vi "02T_WaitForData.vi"(8 "WaitTimeoutMS":u32, 11 "VISA":refnum<visa-resource-name>) -> (0 "Buffer":string, 1 "Bytes at Port":u32, 3 "Data Recived":bool=TRUE)   [LabVIEW 2013]
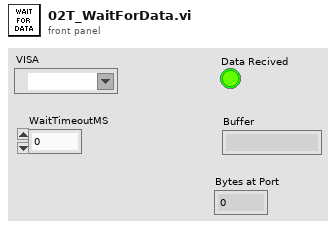
[diagram p1: front panel]
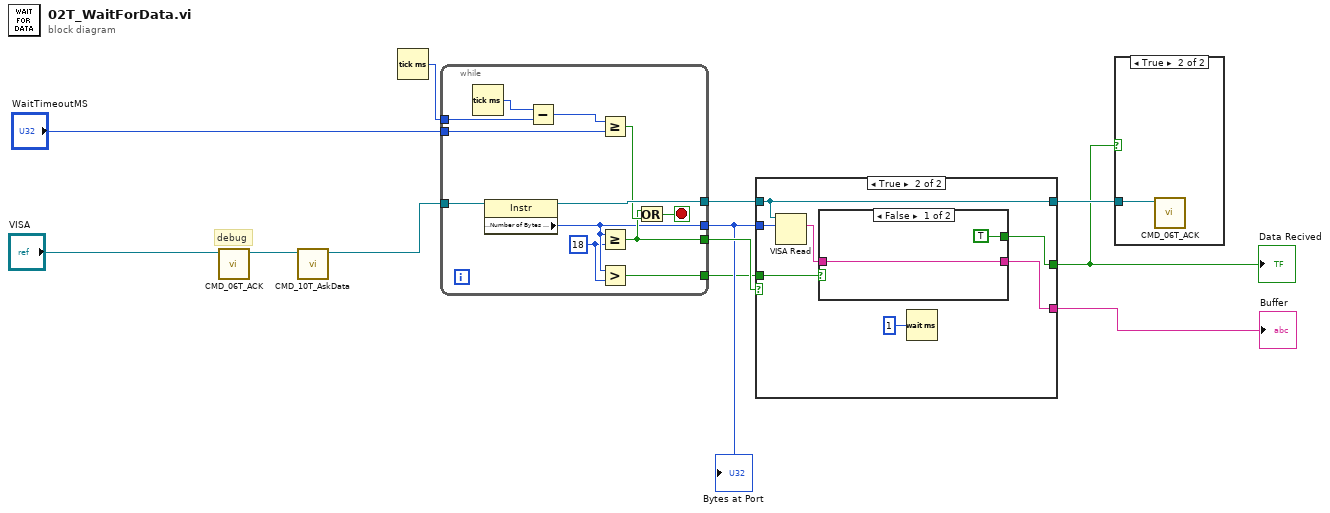
[diagram p0: block diagram]
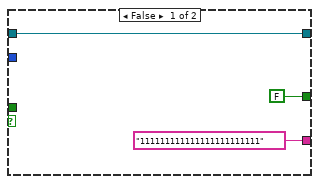
[diagram p3: hidden frame]
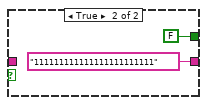
[diagram p4: hidden frame]
diagram:
  # "debug"
  n1 = call "CMD_06T_ACK.vi"("VISA resource name"="VISA") -> ("VISA resource name out"=w1:refnum<visa-resource-name>)  [unwired: 10 in]
  n2 = call "CMD_10T_AskData.vi"("VISA resource name"=w1) -> ("VISA resource name out"=w2:refnum<visa-resource-name>)  [unwired: 10 in]
  n3 = Tick Count (ms)() -> (millisecond timer value=w12:u32)
  n4 = while {
    tunnel: w2 -> [w24]
    tunnel: [w23] -> w9
    tunnel: [w15] -> w8
    tunnel: w12 -> [w20]
    tunnel: "WaitTimeoutMS" -> [w17]
    tunnel: [w16] -> w10
    tunnel: [w13] -> w7
    stop <- w22 stop-if-true
    w14 = u32 18 ("y")
    n5 = Tick Count (ms)() -> (millisecond timer value=w19:u32)
    n6 = property class="Instr"(reference=w24) -> (reference out=w23:refnum<visa-resource-name>, "Serial Settings:Number of Bytes at Serial Port"=w15:u32)  [unwired: 1 in, 1 out]
    n7 = Subtract(x=w19, y=w20) -> (x-y=w18:u32)
    n8 = Greater Or Equal?(x=w18, y=w17) -> (x >= y?=w21:bool)
    n9 = Greater Or Equal?(x=w15, y=w14) -> (x >= y?=w16:bool)
    n10 = Greater?(x=w15, y=w14) -> (0:w13:bool)
    n11 = Or(x=w16, y=w21) -> (x .or. y?=w22:bool)
  }
  "Bytes at Port" <- w8
  n12 = case shown="True" w10 {
    tunnel: w9 -> [w25 w29]
    tunnel: w8 -> [_ w34]
    tunnel: w7 -> [_ w33]
    tunnel: ["111111111111111111111111" ("read buffer") w32] -> w6
    tunnel: [FALSE w30] -> w4
    tunnel: [w25 w29] -> w5
    frame False {
    }
    frame True {
      n13 = VISA Read(VISA resource name=w29, byte count=w34) -> (read buffer=w31:string)  [unwired: 1 in, 3 out]
      n14 = case shown="False" w33 {
        tunnel: [w36 "111111111111111111111111" ("read buffer")] -> w32
        tunnel: w31 -> [w36 _]
        tunnel: [TRUE FALSE] -> w30
        frame False {
        }
        frame True {
        }
      }
      n15 = Wait (ms)(milliseconds to wait=u32 1) -> ()  [unwired: 1 out]
    }
  }
  "Buffer" <- w6
  "Data Recived" <- w4
  n16 = case shown="True" w4 {
    tunnel: w5 -> [_ w39]
    frame False {
    }
    frame True {
      n17 = call "CMD_06T_ACK.vi"("VISA resource name"=w39) -> ()  [unwired: 10 in, 1 out]
    }
  }
